vi "parseElements.vi"(4 "<\"[]\" not present>":bool, 5 "requiredObjectFromPath":string, 6 "Variant":variant, 7 "checkEmptyArrayIndices":bool, 8 "error in (no error)":errorcluster, 9 "jsonString":string, 10 "singlePathElement":string, 11 "checkArraysOrClusters":bool) -> (0 "error out":errorcluster, 2 "VArray":variant, 3 "error?":bool)   [LabVIEW 2015, in "Zen Analytics.lvclass"]
uses:
  Zen Analytics.lvclass
  <vilib>/addons/_JKI.lib/Serialization/JSON/JKI JSON Serialization.lvlib
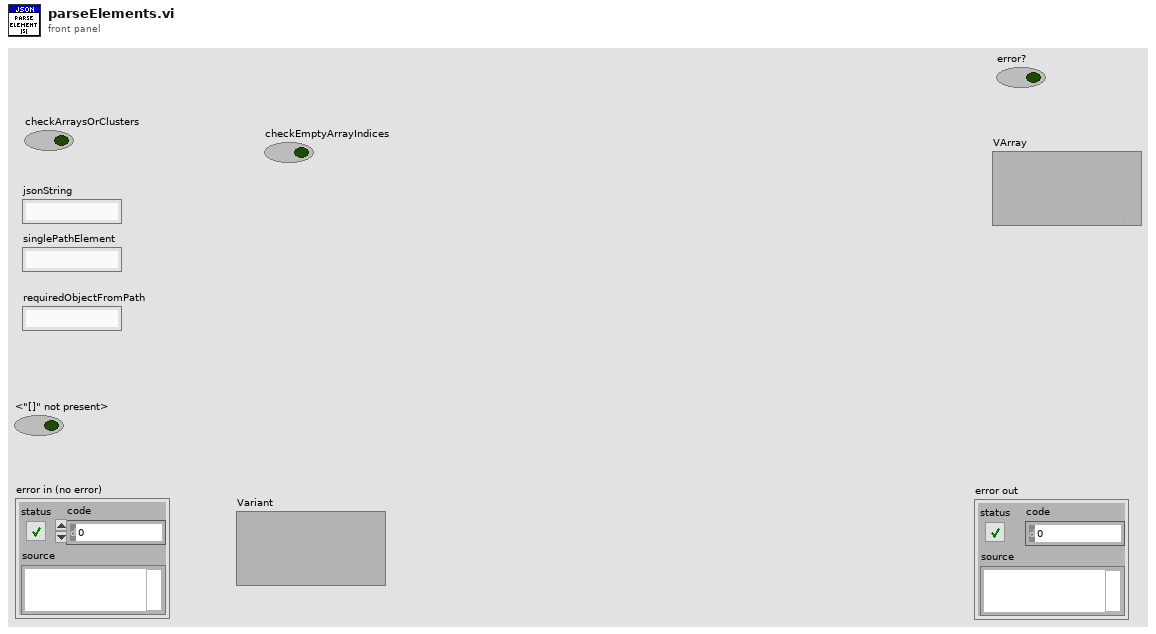
[diagram p1: front panel]
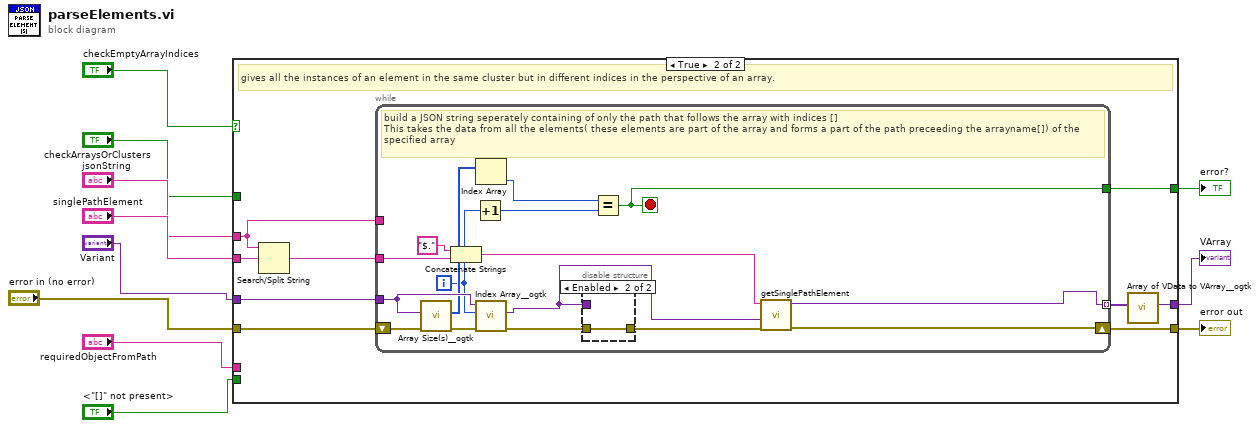
[diagram p0: block diagram]
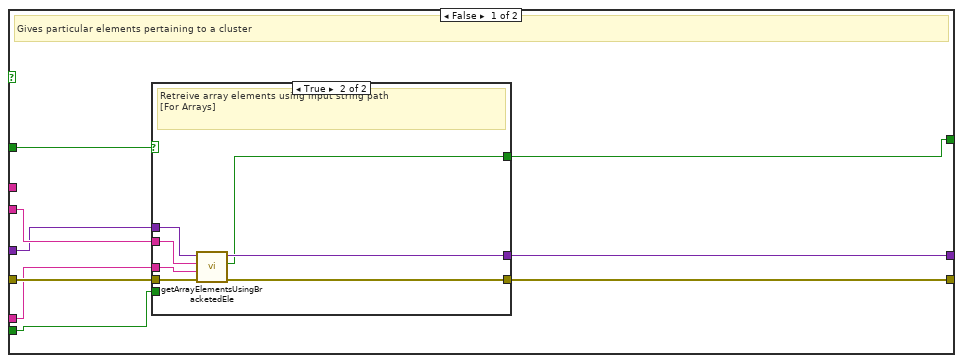
[diagram p2: hidden frame]
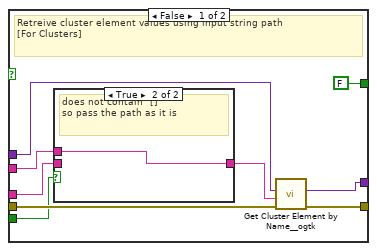
[diagram p3: hidden frame]
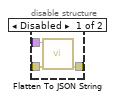
[diagram p5: hidden frame]
diagram:
  n1 = case shown="True" "checkEmptyArrayIndices" {
    tunnel: [w20 w42] -> w7
    tunnel: "error in (no error)" -> [w19 w40]
    tunnel: [w18 w39] -> w2
    tunnel: "requiredObjectFromPath" -> [w17 _]
    tunnel: "singlePathElement" -> [w16 w45]
    tunnel: "checkArraysOrClusters" -> [w15 _]
    tunnel: "<\"[]\" not present>" -> [w14 _]
    tunnel: "Variant" -> [w13 w47]
    tunnel: "jsonString" -> [_ w46]
    tunnel: [w12 w41] -> w11
    frame False {
      # "Gives particular elements pertaining to a cluster"
      n2 = case shown="True" w15 {
        tunnel: w13 -> [w29 w36]
        tunnel: [w28 w38] -> w20
        tunnel: w16 -> [w24 w33]
        tunnel: w19 -> [w27 w34]
        tunnel: [w26 w37] -> w18
        tunnel: w17 -> [w22 w35]
        tunnel: w14 -> [w25 _]
        tunnel: [FALSE ("keygiven?") w32] -> w12
        frame False {
          # "Retreive cluster element values using input string path\n[For Clusters]"
          n3 = case shown="True" w25 {
            tunnel: w24 -> [_ w31]
            tunnel: [w30 w31] -> w23
            tunnel: w22 -> [w30 _]
            frame False {
              # "contains the \"[]\"\nso remove the square brackets"
            }
            frame True {
              # "does not contain \"[]\"\nso pass the path as it is"
            }
          }
          n4 = call <userlib>:"Get Cluster Element by Name__ogtk.vi"("error in (no error)"=w27, "Element Name"=w23, "Cluster"=w29) -> ("error out"=w26:errorcluster, "VElement"=w28:variant)  [unwired: 6 in, 1 out]
        }
        frame True {
          # "Retreive array elements using input string path\n[For Arrays]"
          n5 = call "getArrayElementsUsingBracketedEle.vi"("error in (no error)"=w34, "requriedObject"=w35, "brackettedElements"=w33, "Variant in"=w36) -> ("error out"=w37:errorcluster, "error?"=w32:bool, "Array Element"=w38:variant)  [unwired: 5 in]
        }
      }
    }
    frame True {
      # "gives all the instances of an element in the same cluster but in different indices in the perspective of an array."
      n6 = Search/Split String(string=w46, search string/char (-)=w45) -> (match + rest of string=w44:string)  [unwired: 1 in, 2 out]
      n7 = while {
        tunnel: w47 -> [w63]
        tunnel: w46 -> [_]
        tunnel: w44 -> [w59]
        tunnel: [w50] -> w43 mode=indexing
        tunnel: [w56] -> w41
        shift-right: [w49] -> w39
        shift-left: w40 -> [w55]
        i -> [w58]
        stop <- w56 stop-if-true
        # "build a JSON string seperately containing of only the path that follows the array with indices []\nThis takes the data from all the elements( these elements are part of the array and forms a part of the path preceeding the arrayname[]) of the specified array"
        n8 = call <userlib>:"Array Size(s)__ogtk.vi"("error in (no error)"=w55, "Array"=w63) -> ("error out"=w54:errorcluster, "Size(s)"=w62:u32[])  [unwired: 7 in, 1 out]
        n9 = Concatenate Strings("$." ("string"), w59) -> (w51:string)
        n10 = Increment(x=w58) -> (x+1=w57:i32)
        n11 = Index Array(array=w62) -> (element=w61:u32)  [unwired: 1 in]
        n12 = call <userlib>:"Index Array__ogtk.vi"("error in (no error)"=w54, "Index (1D)"=w58, "MultiD Array"=w63) -> ("error out"=w53:errorcluster, "Array Element"=w48:variant)  [unwired: 7 in]
        n13 = disable-structure shown="Enabled" {
          disable-tunnel: w53 -> [w66 w67]
          disable-tunnel: [w65 w67] -> w52
          disable-tunnel: w48 -> [w64 _]
          frame Disabled {
            n14 = call <vilib>:"Flatten To JSON String.vi"("error in (no error)"=w66, "Variant"=w64) -> ("error out"=w65:errorcluster)  [unwired: 8 in, 1 out]
          }
          frame Enabled {
          }
        }
        n15 = Equal?(x=w61, y=w57) -> (x = y?=w56:bool)
        n16 = call "getSinglePathElement.vi"("error in (no error)"=w52, "Variant in"=w48, "String"=w51) -> ("error out"=w49:errorcluster, "Variant out"=w50:variant)  [unwired: 7 in]
      }
      n17 = call <userlib>:"Array of VData to VArray__ogtk.vi"("1D Array of VData"=w43) -> ("VArray"=w42:variant)  [unwired: 9 in, 1 out]
    }
  }
  "error?" <- w11
  "VArray" <- w7
  "error out" <- w2
